vi "XML_FF_openToWrite.vi"() -> (0 "error out":errorcluster, 3 "DOM document out":refnum<k20>)   [LabVIEW 2016, in "XML_EEG_Features.lvlib"]
uses:
  XML_EEG_Features.lvlib
  <vilib>/xml/NI_XML.lvlib
  <resource>/objmgr/DOMUserDefRef.rc
panel:
  # "This VI is a part of BCI Design library, http://www.ru-bci.org \nCopyright © 2020, Sotnikov Peter, All rights reserved. License: CC BY-NC 4.0"
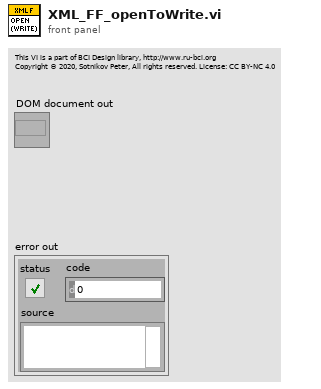
[diagram p1: front panel]
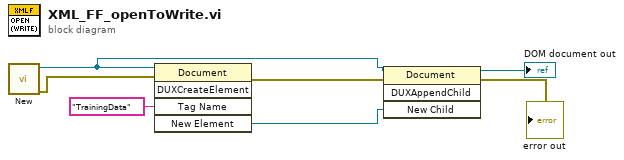
[diagram p0: block diagram]
diagram:
  n1 = call <vilib>:"New.vi"() -> ("error out"=w6:errorcluster, "DOM document out"=w5:refnum<k20>)  [unwired: 8 in]
  n2 = invoke class="Document" method="DUXCreateElement"(reference=w5, error in=w6, "Tag Name"="TrainingData") -> (error out=w3:errorcluster, "New Element"=w4:refnum<k20>)  [unwired: 2 in, 3 out]
  n3 = invoke class="Document" method="DUXAppendChild"(reference=w5, error in=w3, "New Child"=w4) -> (reference out=→"DOM document out":refnum<k20>, error out=→"error out":errorcluster)  [unwired: 1 in, 2 out]
